vi "SysIDRealtime2.vi"() -> ()   [LabVIEW 2011, in "SysIDRealtime.lvlib"]
doc: "This VI was generated automatically using the FPGA Wizard. You can modify the VI normally."
uses:
  SysIDRealtime.lvlib
  <vilib>/Platform/TimedLoop/XDataNode/timing_clust.ctl
  <vilib>/Platform/TimedLoop/XDataNode/nitl_modes.ctl
  <vilib>/Platform/TimedLoop/XDataNode/wakeup.ctl
  <vilib>/FPGAPlugInAG/sbRIO-9632/niLvFpga_Open_sbRIO-9632.vi
  <vilib>/rvi/interface/common/dynamic/niFpgaDynamicAddResources.vi
  <vilib>/FPGAPlugInAG/Dynamic/niLvFpga_Reset_Dynamic.vi
  <vilib>/FPGAPlugInAG/Dynamic/niLvFpga_Run_Dynamic.vi
  <vilib>/Utility/error.llb/Error Cluster From Error Code.vi
  <vilib>/rvi/errors/niLvFpgaAdjustHostInterfaceError.vi
  <vilib>/FPGAPlugInAG/Dynamic/niLvFpga_Close_Dynamic.vi
  <vilib>/rvi/interface/nirviOpenFPGA/nirviOpenFPGA.xnode
  FPGA Bitfiles/PPDControlLab3_FPGA_IP8.lvbitx
  <vilib>/rvi/interface/nirviMethod/nirviMethod.xnode
  <vilib>/Platform/TimedLoop/XDataNode/XDataNode.xnode
  <vilib>/rvi/interface/nirviReadWriteControl/nirviReadWriteControl.xnode
  <vilib>/rvi/interface/nirviCloseFPGA/nirviCloseFPGA.xnode
  <vilib>/rvi/interface/Simulation/niFpgaSimulationCallBeginRW.vi
  NiFpgaLv.dll
  <vilib>/Platform/TimedLoop/XDataNode/XDNodeRunTimeDep.lvlib
  <vilib>/Analysis/NI_AALBase.lvlib
panel:
  out "Amp In":dbl[](graph)
  out "Amp Cpmmand":fxp<+/-,20,5>
  out "Iteration Duration":i64
  out "Position":i32[](graph)
  in  "Control Rate (ticks)":u32=800
  out "error":i32
  out "Waveform Graph":i32[](graph)
  in  "f2":dbl=0.5 format="%0.2f"
  in  "f1":dbl=0.001
  in  "amplitude":dbl=16384.0 format="%0.2f"
  in  "Period (us)":i64=15000
  out "Finished Late? [i-1]":bool
  out "quad saved (Port0/DIO0,Port0/DIO1)":cluster{"Position":i32, "Index Count":u16}
  out "quad pos (Port0/DIO0,Port0/DIO1)":i32
  in  "AO (ModB/AO2)":fxp<+/-,20,5>
  in  "AO (ModB/AO1)":fxp<+/-,20,5>
  out "AI (ModA/AI0)":fxp<+/-,26,5> format="%.6g"
  out "Late? Latched":bool
  in  "Local Stop 0":bool
  in  "Start 0":bool
  in  "Loop Rate (Hz)":dbl=100000.0
  out "Calculated Rate (Hz)":dbl
  out "error out":errorcluster
  in  "Global Stop":bool
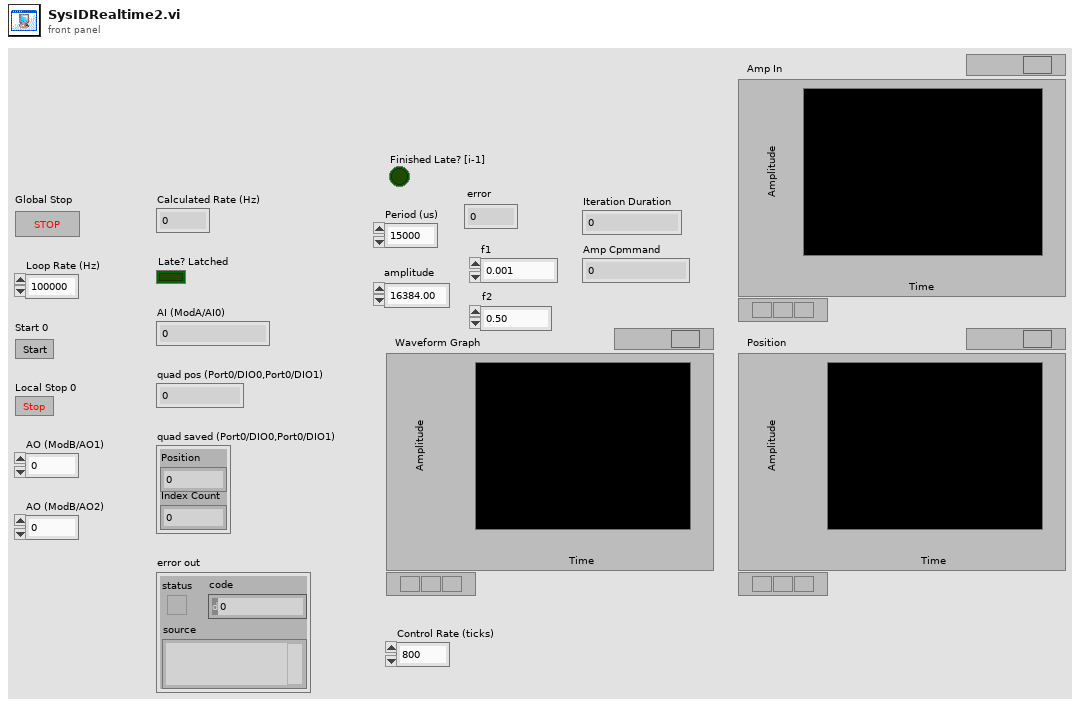
[diagram p1: front panel]
types:
  T1 = typedef "XDNodeRunTimeDep.lvlib/timing_clust.ctl" = cluster{"Expected End [f-1]":u64, "Actual End [f-1]":u64, "Finished Late? [f-1]":bool, "Expected End [i-1]":u64, "Actual End [i-1]":u64, "Finished Late? [i-1]":bool, "Expected Start [i]":u64, "Actual Start [i]":u64, "Expected Start [f]":u64, "Actual Start [f]":u64, "Source Name":string, "Structure Name":string, "Period":i64, "Deadline":i64, "Offset":i64, "Start":i64, "Priority":i32, "Timeout":i32, "Mode":T2, "Wakeup Reason":T3, "Error":errorcluster, "Source Type":string, "Secondary Source Type":string, "Global End Time":u64, "Global Start Time":u64, "Frame Duration":u64, "Iteration Duration":u64, "Assigned CPU":i32, "I/O Scan Engine Mode":u32}
  T2 = typedef "XDNodeRunTimeDep.lvlib/nitl_modes.ctl" = enum32{"No Change", "Process missed periods, maintain original phase", "Discard missed periods, maintain original phase", "Process missed periods, ignore original phase", "Discard missed periods, ignore original phase"}
  T3 = typedef "XDNodeRunTimeDep.lvlib/wakeup.ctl" = enum32{"Normal", "Aborted", "Asynchronous wakeup", "Timing source error", "Timed loop error", "Timeout"}
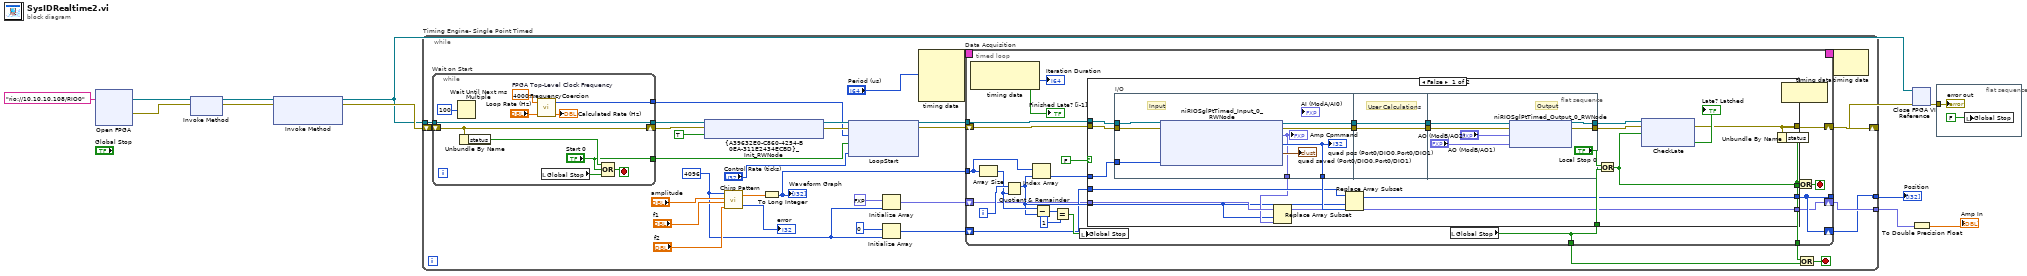
[diagram p0: block diagram]
diagram:
  n1 = xnode ("Open FPGA")("resource name"=tag "rio://10.10.10.108/RIO0") -> ("FPGA VI Reference Out"=w7:refnum<k20>, "error out"=w8:errorcluster)  [unwired: 1 in]
  n2 = xnode ("Invoke Method")("FPGA VI Reference In"=w7, "error in"=w8) -> ("FPGA VI Reference Out"=w11:refnum<k20>, "error out"=w12:errorcluster)
  n3 = xnode ("Invoke Method")("FPGA VI Reference In"=w11, "error in"=w12) -> ("FPGA VI Reference Out"=w9:refnum<k20>, "error out"=w10:errorcluster)  [unwired: 1 in]
  n4 = while "Timing Engine- Single Point Timed" {
    tunnel: w9 -> [w41]
    shift-right: [w40] -> w6
    shift-left: w10 -> [w44]
    tunnel: [w13] -> w4
    tunnel: [w14] -> w3
    stop <- w35 stop-if-true
    w16 = 4096 ("samples")
    n5 = while "Wait on Start" {
      tunnel: w41 -> [w123]
      tunnel: [w123] -> w39
      tunnel: [w115] -> w32
      tunnel: ["Start 0"] -> w31
      shift-right: [w117] -> w38
      shift-left: w44 -> [w117]
      stop <- w124 stop-if-true
      w118 = 40000000.0  # FPGA Top-Level Clock Frequency
      n6 = Wait Until Next ms Multiple(millisecond multiple=u32 100) -> ()  [unwired: 1 out]
      n7 = Unbundle By Name(w117) -> ("status"=w116:bool)
      n8 = call "FrequencyCoercion.vi"("Loop Rate (Hz)"="Loop Rate (Hz)", "FPGA Top-Level Clock Frequency"=w118) -> ("Actual Rate (Hz)"=→"Calculated Rate (Hz)":dbl, "FPGA Ticks"=w115:u32)  [unwired: 2 in]
      n9 = local read "Global Stop"() -> (w121:bool)
      n10 = Compound Arithmetic op=OR(w116, "Start 0", w121) -> (w124:bool)
    }
    n11 = xnode ("{A39632E0-C860-4254-B0EA-311E2434ECBD}_Init_RWNode")("FPGA VI Reference In"=w39, "error in"=w38, "quad reset (Port0/DIO0,Port0/DIO1)"=TRUE ("const")) -> ("FPGA VI Reference Out"=w33:refnum<k20>, "error out"=w37:errorcluster)
    n12 = call <vilib>:"Chirp Pattern.vi"("f2"="f2", "f1"="f1", "amplitude"="amplitude", "samples"=w16) -> ("error"=→"error":i32, "Chirp Pattern"=w22:dbl[])
    n13 = To Long Integer(number=w22) -> (32bit integer=w21:i32[])
    "Waveform Graph" <- w21
    n14 = xnode ("LoopStart")("FPGA VI Reference In"=w33, "error in"=w37, "Loop Rate (Ticks)"=w32, "Start 0"=w31, "Control Rate (ticks)"="Control Rate (ticks)") -> ("FPGA VI Reference Out"=w43:refnum<k20>, "error out"=w42:errorcluster)
    n15 = Initialize Array(0 ("quad pos (Port0/DIO0,Port0/DIO1)"), w16) -> (w18:i32[])
    n16 = Initialize Array(fxp<+/-,20,5> 0.0 ("Amp Cpmmand"), w16) -> (w15:fxp<+/-,20,5>[])
    n17 = node-c288("Period (us)") -> (w29:T1)  [unwired: 3 in]
    n18 = timed-loop "Data Acquisition" {
      tunnel: w43 -> [w61]
      tunnel: [w63] -> w36
      tunnel: [w62] -> w34
      shift-right: [w66] -> w40
      shift-left: w42 -> [w60]
      timing: w29 -> [_]
      timing-out: [_] -> w28
      tunnel: w21 -> [w56]
      tunnel: [w46] -> _
      shift-right: [w45] -> w14
      shift-left: w15 -> [w47]
      shift-right: [w46] -> w13
      shift-left: w18 -> [w49]
      i -> [w57]
      stop <- w64 stop-if-true
      n19 = node-c288() -> (→"Finished Late? [i-1]":bool, →"Iteration Duration":i64)  [unwired: 1 in]
      n20 = Array Size(array=w56) -> (size(s)=w54:i32)
      n21 = Quotient & Remainder(x=w57, y=w54) -> (x-y*floor(x/y)=w50:i32)  [unwired: 1 out]
      n22 = Index Array(array=w56, index=w50) -> (element=w55:i32)
      n23 = Subtract(x=w54, y=w50) -> (x-y=w53:i32)
      n24 = Equal?(x=w53, y=1) -> (x = y?=w51:bool)
      n25 = local write "Global Stop"(w51) -> ()
      n26 = local read "Global Stop"() -> (w63:bool)
      n27 = case "Timeout" shown="False" FALSE {
        tunnel: w61 -> [w86 _]
        tunnel: w60 -> [w85 w109]
        tunnel: [w79 w109] -> w66
        tunnel: [w81 w108] -> w65
        tunnel: w63 -> [w82 w108]
        tunnel: w55 -> [w78 _]
        tunnel: w50 -> [w72 _]
        tunnel: w49 -> [w76 _]
        tunnel: [w75 _] -> w46
        tunnel: w47 -> [w74 _]
        tunnel: [w71 _] -> w45
        frame False {
          n28 = flat-sequence "I/O" {
            tunnel: w86 -> [w97]
            tunnel: w85 -> [w99]
            tunnel: [w98] -> w91
            tunnel: [w96] -> w88
            tunnel: w78 -> [w94]
            tunnel: [w93] -> w77
            tunnel: [w92] -> w73
            tunnel: [w101] -> w90
            tunnel: w91 -> [w100]
            tunnel: w88 -> [w101]
            tunnel: [w100] -> w89
            tunnel: [w106] -> w84
            tunnel: [w104] -> w87
            tunnel: w90 -> [w105]
            tunnel: w89 -> [w107]
            frame #0 {
              # "Input"
              n29 = xnode ("niRIOSglPtTimed_Input_0_RWNode")("FPGA VI Reference In"=w97, "error in"=w99, "Reference"=w94) -> ("FPGA VI Reference Out"=w96:refnum<k20>, "error out"=w98:errorcluster, "Amp Cpmmand"=w92:fxp<+/-,20,5>, "quad pos (Port0/DIO0,Port0/DIO1)"=w93:i32, "quad saved (Port0/DIO0,Port0/DIO1)"=→"quad saved (Port0/DIO0,Port0/DIO1)":cluster{"Position":i32, "Index Count":u16})
              "quad pos (Port0/DIO0,Port0/DIO1)" <- w93
              "Amp Cpmmand" <- w92
            }
            frame #1 {
              # "User Calculations"
            }
            frame #2 {
              # "Output"
              n30 = xnode ("niRIOSglPtTimed_Output_0_RWNode")("FPGA VI Reference In"=w105, "error in"=w107, "AO (ModB/AO1)"="AO (ModB/AO1)", "AO (ModB/AO2)"="AO (ModB/AO2)") -> ("FPGA VI Reference Out"=w104:refnum<k20>, "error out"=w106:errorcluster)
            }
          }
          n31 = Replace Array Subset(array=w74, new element=w73, index=w72) -> (w71:fxp<+/-,20,5>[])
          n32 = Replace Array Subset(array=w76, new element=w77, index=w72) -> (w75:i32[])
          n33 = Or(x="Local Stop 0", y=w82) -> (x .or. y?=w81:bool)
          n34 = xnode ("CheckLate")("FPGA VI Reference In"=w87, "error in"=w84, "Local Stop 0"=w81) -> ("error out"=w79:errorcluster, "Late? Latched"=→"Late? Latched":bool)  [unwired: 1 out]
        }
        frame True {
          # "Timeout waiting for an interrupt. This case checks the state of the global stop.\nIf global stop is not set, then loop around to wait for an interrupt again."
        }
      }
      n35 = Unbundle By Name(w66) -> ("status"=w62:bool)
      n36 = node-c288() -> ()  [unwired: 1 in, 1 out]
      n37 = Or(x=w62, y=w65) -> (x .or. y?=w64:bool)
    }
    n38 = Or(x=w34, y=w36) -> (x .or. y?=w35:bool)
    n39 = node-c288(w28) -> ()  [unwired: 1 out]
  }
  "Position" <- w4
  n40 = xnode ("Close FPGA VI Reference")("FPGA VI Reference In"=w9, "error in"=w6) -> ("error out"=w5:errorcluster)
  n41 = To Double Precision Float(number=w3) -> (double precision float=→"Amp In":dbl[])
  n42 = flat-sequence {
    tunnel: w5 -> [w126]
    frame #0 {
      n43 = local write "Global Stop"(FALSE ("Global Stop")) -> ()
      "error out" <- w126
    }
  }
